vi "uActor_Send_Stop_Synchronous.vi"(8 "error in (no error)":errorcluster, 11 "uActor Transport":refnum<class "uTransport_uActor.lvclass">) -> (0 "error out":errorcluster)   [LabVIEW 2023, in "uLib.lvlib" / "uActor.lvclass"]
doc: "Send a STOP message to the actor and block dataflow until verifying that the actor had shutdown.\nThis methods executes regardless of incoming errors."
uses:
  uActor.lvclass
  uTransport/uTransport_uActor/uTransport_uActor.lvclass
  uMsg/uMsg/uMsg.lvclass/uMsg.ctl
  uTransport/uTransport_uActor/uTransport_uActor.lvclass/uTransport_uActor.ctl
  uActor_CMDs_Prefix.vi
  uActor_SimpleSend.vi
  uActor_SendMsg.vi
  uMsg/uMsg/uMsg Create.vi
  uTransport/uTransport_uActor/uTransport_uActor_SendMsg.vi
  uMsg/uMsg/uMsg Update Timestamp.vi
  uData/uData/uData.lvclass
  uTransport/uTransport/uTransport.lvclass
  uMsg/uMsg/uMsg.lvclass
  uActor.lvclass/uActor.ctl
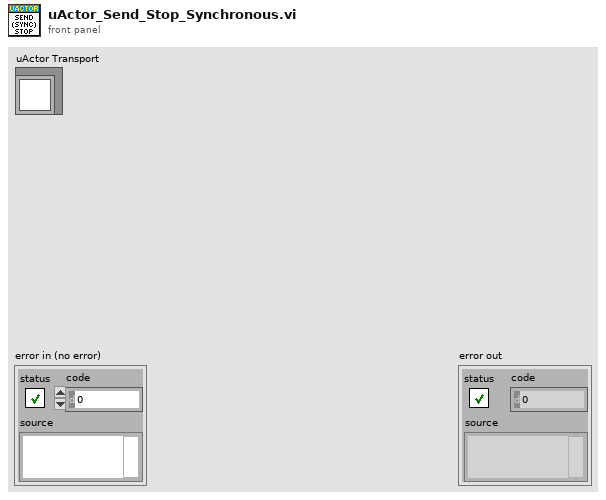
[diagram p1: front panel]
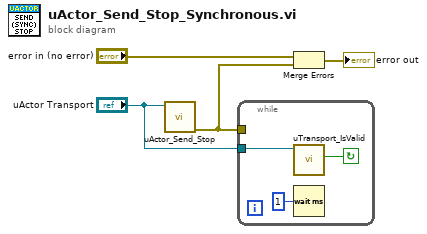
[diagram p0: block diagram]
diagram:
  n1 = call "uActor_Send_Stop.vi"("uActor Transport"="uActor Transport") -> ("error out"=w2:errorcluster)  [unwired: 10 in]
  n2 = while {
    tunnel: w2 -> [_]
    tunnel: "uActor Transport" -> [w7]
    stop <- w6 continue-if-true
    n3 = call-dynamic "uTransport_IsValid.vi"("uTransport_uActor in"=w7) -> ("IsValid?"=w6:bool)  [unwired: 8 in, 2 out]
    n4 = Wait (ms)(milliseconds to wait=u32 1) -> ()  [unwired: 1 out]
  }
  n5 = Merge Errors("error in (no error)", w2) -> (→"error out":errorcluster)
